vi "DictToArray.vi"(8 "entrée d'erreur (pas d'erreur)":errorcluster, 11 "Dict":string) -> (0 "sortie d'erreur":errorcluster, 3 "String 2DArray":string[][](array[string]))   [LabVIEW 2020]
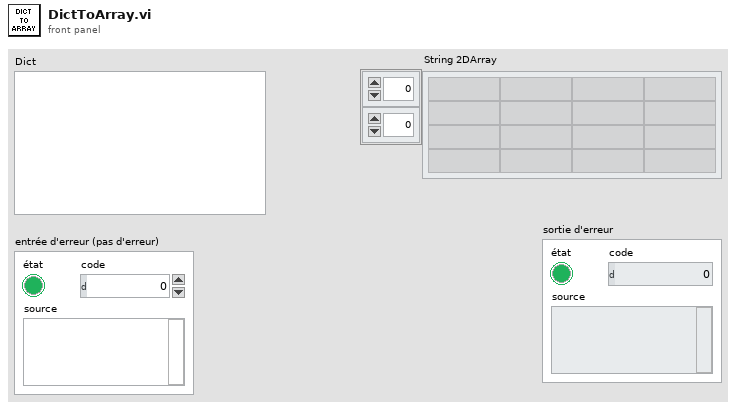
[diagram p1: front panel]
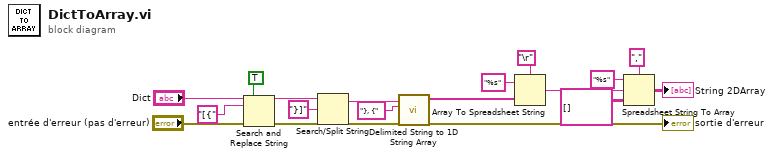
[diagram p0: block diagram]
diagram:
  n1 = Search and Replace String(replace all?=TRUE ("replace all? (F)"), input string="Dict", search string="[{", error in="entrée d'erreur (pas d'erreur)") -> (result string=w4:string, error out=→"sortie d'erreur":errorcluster)  [unwired: 4 in, 2 out]
  n2 = Search/Split String(string=w4, search string/char (-)="}]" ("chaîne/car. recherché (-)")) -> (substring before match=w11:string)  [unwired: 1 in, 2 out]
  n3 = call <vilib>:"Delimited String to 1D String Array.vi"("delimiter"="}, {", "delimited string"=w11) -> ("string array"=w13:string[])  [unwired: 9 in]
  n4 = Array To Spreadsheet String(delimiter (Tab)="\r", array=w13, 3:"%s" ("chaîne de format")) -> (spreadsheet string=w5:string)
  n5 = Spreadsheet String To Array(delimiter (Tab)="," ("séparateur (Tabulation)"), format string="%s" ("chaîne de format"), spreadsheet string=w5, array type (2D Dbl)=string[][] []) -> (array=→"String 2DArray":string[][])
